vi "merFISH_convert_laser_lines_array_for_FPGA.vi"(3 "Laser lines array":dbl[][](array[numeric])) -> (0 "Laser power":sgl[](array[numeric]), 1 "Laser lines":i32[](array[numeric]))   [LabVIEW 2015]
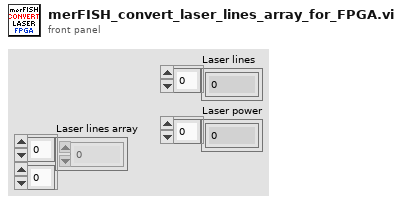
[diagram p1: front panel]
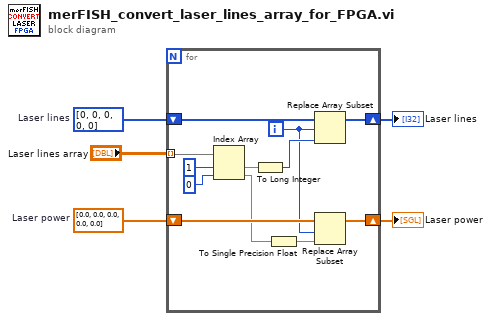
[diagram p0: block diagram]
diagram:
  w3 = sgl[] [0.0, 0.0, 0.0, 0.0, 0.0]  # Laser power
  w4 = i32[] [0, 0, 0, 0, 0]  # Laser lines
  n1 = for {
    tunnel: "Laser lines array" -> [w15] mode=indexing
    shift-right: [w11] -> w2
    shift-left: w4 -> [w12]
    shift-right: [w6] -> w1
    shift-left: w3 -> [w10]
    i -> [w9]
    n2 = Index Array(array=w15, index #1=1 ("index"), index #2=0 ("index")) -> (element #1=w14:dbl, element #2=w8:dbl)
    n3 = To Long Integer(number=w14) -> (32bit integer=w13:i32)
    n4 = To Single Precision Float(number=w8) -> (single precision float=w7:sgl)
    n5 = Replace Array Subset(array=w12, new element=w13, index=w9) -> (w11:i32[])
    n6 = Replace Array Subset(array=w10, new element=w7, index=w9) -> (w6:sgl[])
  }
  "Laser lines" <- w2
  "Laser power" <- w1
